vi "Sequence.Test.DMC.GetDMCSize.vi"() -> (1 "max size":i32)   [LabVIEW 2016]
uses:
  Drivers/V7310/LowLevel/V7310.Global.vi
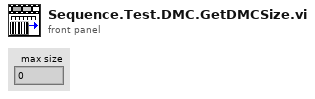
[diagram p1: front panel]
types:
  T1 = typedef "V7310.Data.Status.ctl" = cluster{"State":T2, "LaserStatus":T3, "LaserStatusRaw":string, "Ref":refnum<k5>, "RTC TS":timestamp, "Conn TS":timestamp, "Msg":T4[], "JobInUse":string, "Jobs":string[], "Vars":T5[]}
  T2 = typedef "V7310.Data.Status.State.ctl" = enum16{"First", "Init", "Msg", "Error", "Abort", "Idle", "Run"}
  T3 = typedef "V7310.LaserStatus.ctl" = enum16{"-", "FatalError", "Initialize", "KeySwitchOpen", "TimeoutInterlock", "InterlockOpen", "StartUp", "ShutterlockOpen", "Standby", "Ready", "PrepareForMarking", "WaitForTrigger", "Marking"}
  T4 = typedef "V7310.Message.Data.ctl" = cluster{"ID":i32, "Msg":string}
  T5 = typedef "V7310.Job.Variable.ctl" = cluster{"Name":string, "Value":string}
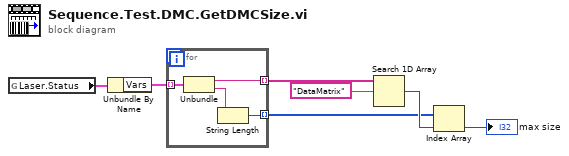
[diagram p0: block diagram]
diagram:
  n1 = global read "V7310.Global.vi" "Laser.Status"() -> (w6:T1)
  n2 = Unbundle By Name(w6) -> ("Vars"=w5:T5[])
  n3 = for {
    tunnel: w5 -> [w11] mode=indexing
    tunnel: [w10] -> w3 mode=indexing
    tunnel: [w8] -> w2 mode=indexing
    n4 = Unbundle(w11) -> ("Name"=w10:string, "Value"=w9:string)
    n5 = String Length(string=w9) -> (length=w8:i32)
  }
  n6 = Search 1D Array(1D array=w3, element="DataMatrix") -> (index of element=w4:i32)  [unwired: 1 in]
  n7 = Index Array(array=w2, index=w4) -> (element=→"max size":i32)
